vi "AD（V3.2）150M.vi"(2 "量程选择":u32, 8 "N-length":dbl, 9 "M-length":dbl, 10 "hDevice":i32, 11 "待读取数据长度":u32) -> (0 "幅频谱":dbl[](graph), 1 "时域谱":dbl[](graph), 3 "hDevice out":i32)   [LabVIEW 2016]
uses:
  <vilib>/Analysis/2dsp.llb/Real FFT.vi
  <vilib>/Analysis/NI_AALPro.lvlib
  E:/PCI8552B/Driver/INF/Win32&Win64/amd64/PCI8552B_32.dll
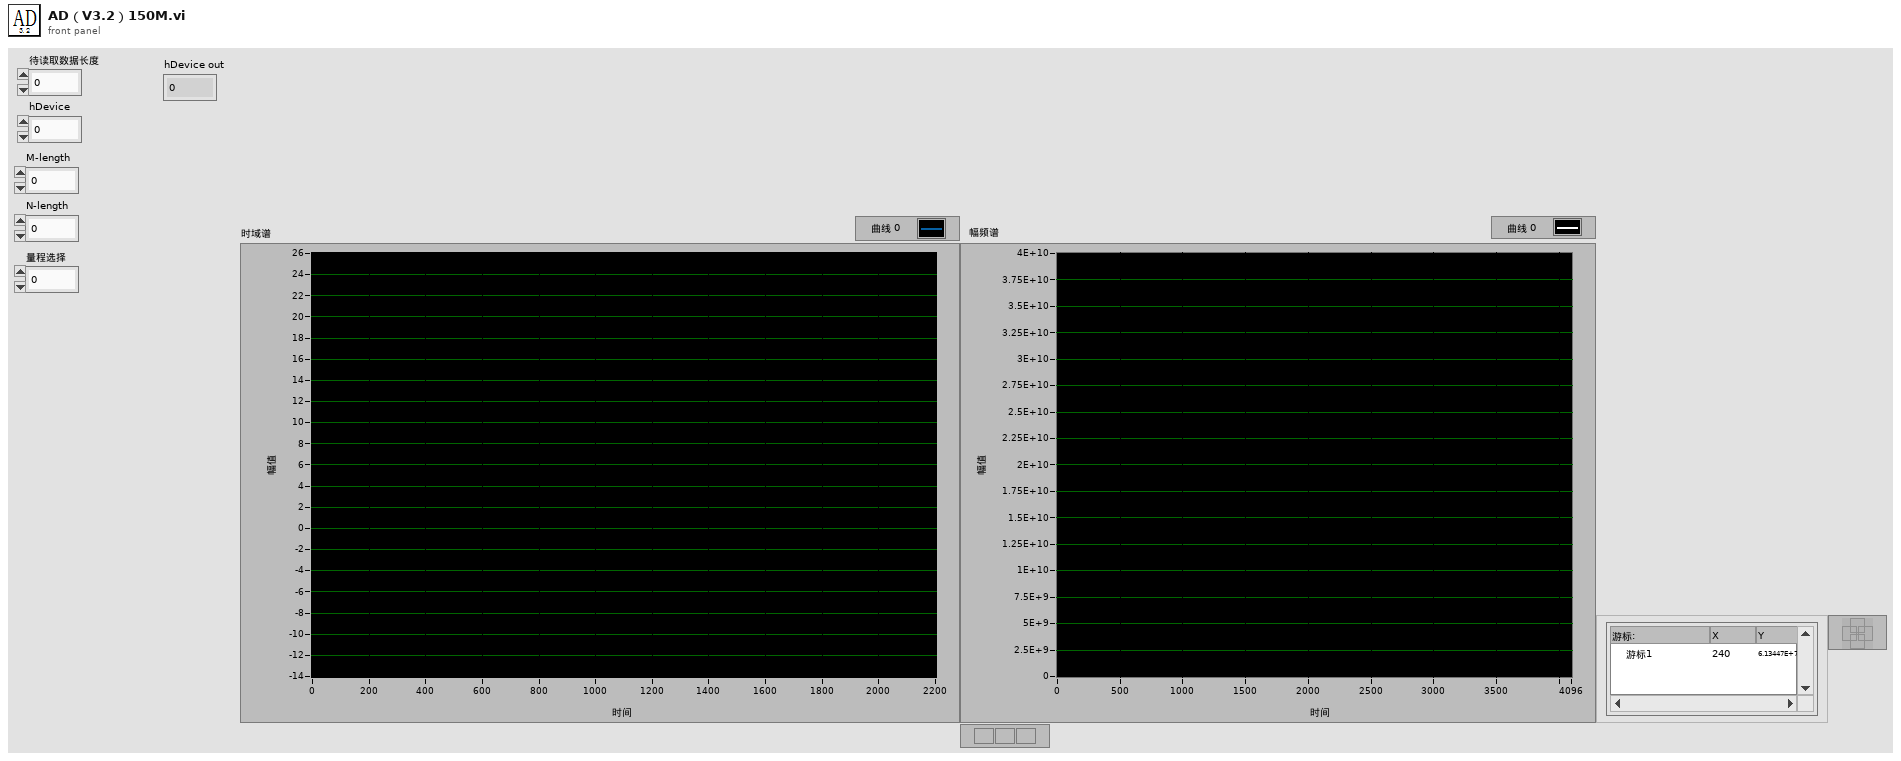
[diagram p1: front panel]
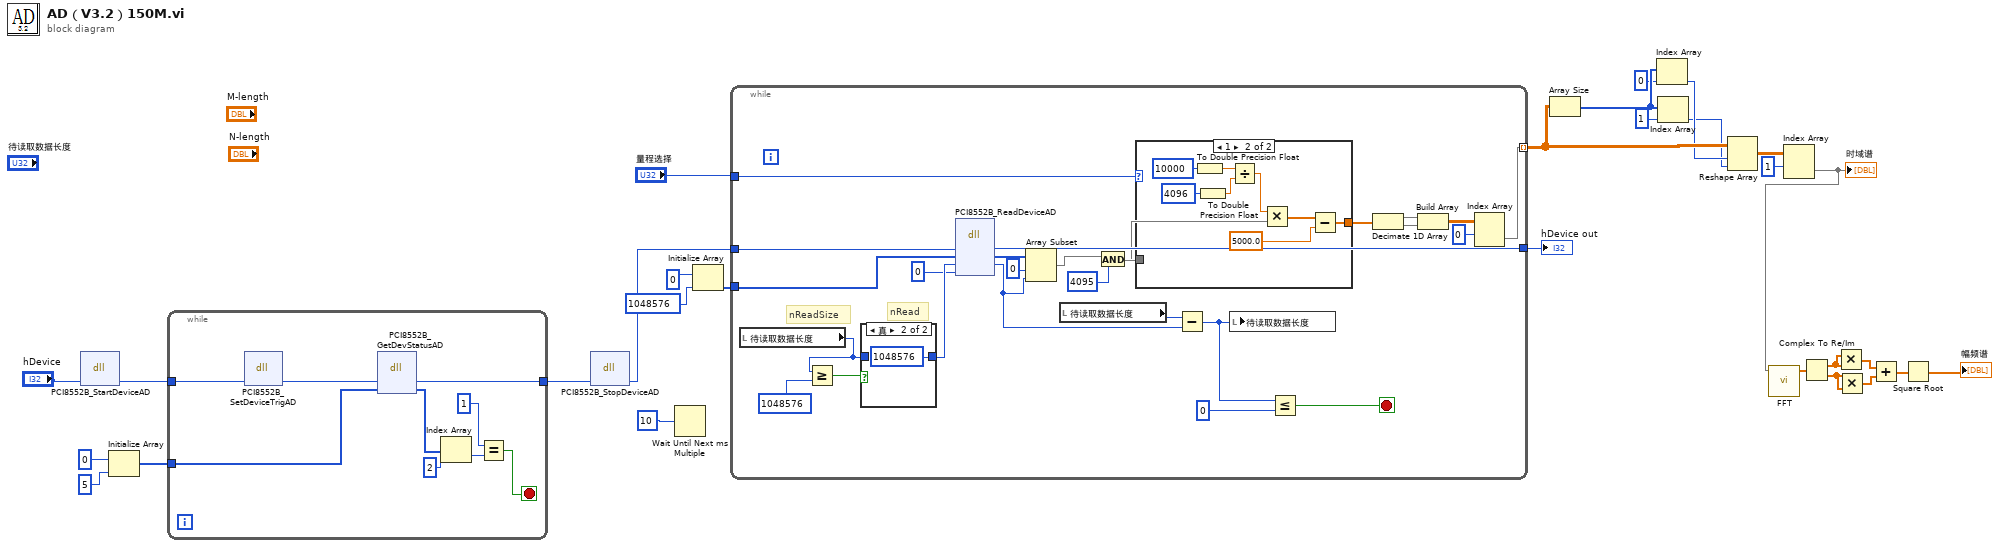
[diagram p0: block diagram]
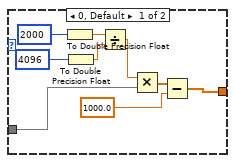
[diagram p2: hidden frame]
diagram:
  n1 = dll-call lib="E:/PCI8552B/Driver/INF/Win32&Win64/amd64/PCI8552B_32.dll" fn="PCI8552B_StartDeviceAD" label="StartDeviceAD"("hDevice"="hDevice") -> ("hDevice"=w24:i32)  [unwired: 4 in, 2 out]
  n2 = Initialize Array(0, 5) -> (w28:i32[])
  n3 = while {
    tunnel: w24 -> [w34]
    tunnel: w28 -> [w38]
    tunnel: [w32] -> w25
    stop <- w31 stop-if-true
    n4 = dll-call lib="E:/PCI8552B/Driver/INF/Win32&Win64/amd64/PCI8552B_32.dll" fn="PCI8552B_SetDeviceTrigAD" label="SetDeviceTrigAD"("hDevice"=w34) -> ("hDevice"=w33:i32)  [unwired: 4 in, 2 out]
    n5 = dll-call lib="E:/PCI8552B/Driver/INF/Win32&Win64/amd64/PCI8552B_32.dll" fn="PCI8552B_GetDevStatusAD" label="GetDevStatusAD"("hDevice"=w33, "ADStatus"=w38) -> ("hDevice"=w32:i32, "ADStatus"=w35:i32[])  [unwired: 4 in, 2 out]
    n6 = Index Array(array=w35, index=2) -> (element=w30:i32)
    n7 = Equal?(x=1, y=w30) -> (x = y?=w31:bool)
  }
  n8 = dll-call lib="E:/PCI8552B/Driver/INF/Win32&Win64/amd64/PCI8552B_32.dll" fn="PCI8552B_StopDeviceAD" label="StopDeviceAD"("hDevice"=w25) -> ("hDevice"=w20:i32)  [unwired: 4 in, 2 out]
  n9 = Wait Until Next ms Multiple(millisecond multiple=u32 10) -> ()  [unwired: 1 out]
  n10 = Initialize Array(u16 0 ("y"), 1048576 ("y")) -> (w21:u16[])
  n11 = while {
    tunnel: w20 -> [w63]
    tunnel: [w62] -> w10
    tunnel: w21 -> [w61]
    tunnel: "量程选择" -> [w51]
    tunnel: [w39] -> w9 mode=indexing
    stop <- w42 stop-if-true
    # "nReadSize"
    # "nRead"
    n12 = local read "待读取数据长度"() -> (w57:u32)
    n13 = Greater Or Equal?(x=w57, y=1048576 ("millisecond multiple")) -> (x >= y?=w59:bool)
    n14 = case shown="真" w59 {
      tunnel: [w82 1048576 ("millisecond multiple")] -> w54
      tunnel: w57 -> [w82 _]
      frame False {
      }
      frame True {
      }
    }
    n15 = dll-call lib="E:/PCI8552B/Driver/INF/Win32&Win64/amd64/PCI8552B_32.dll" fn="PCI8552B_ReadDeviceAD" label="ReadDeviceAD"("hDevice"=w63, "pADBuffer"=w61, "nReadSizeWords"=w54, "nRetSizeWords"=0) -> ("hDevice"=w62:i32, "pADBuffer"=w48:u16[], "nReadSizeWords"=w45:u32)  [unwired: 5 in, 2 out]
    n16 = Array Subset(array=w48, index=0 ("索引"), length=w45) -> (w47:u16[])
    n17 = local read "待读取数据长度"() -> (w56:u32)
    n18 = And(x=w47, y=u16 4095) -> (x .and. y?=w52:u16[])
    n19 = case shown="1" w51 {
      tunnel: w52 -> [w71 w76]
      tunnel: [w64 w75] -> w50
      frame 0, Default {
        n20 = To Double Precision Float(number=2000 ("x")) -> (double precision float=w67:dbl)
        n21 = To Double Precision Float(number=4096) -> (double precision float=w66:dbl)
        n22 = Divide(x=w67, y=w66) -> (x/y=w72:dbl)
        n23 = Multiply(x=w72, y=w71) -> (x*y=w70:dbl[])
        n24 = Subtract(x=w70, y=1000.0) -> (x-y=w64:dbl[])
      }
      frame 1 {
        n25 = To Double Precision Float(number=10000 ("x")) -> (double precision float=w74:dbl)
        n26 = To Double Precision Float(number=4096) -> (double precision float=w78:dbl)
        n27 = Divide(x=w74, y=w78) -> (x/y=w81:dbl)
        n28 = Multiply(x=w81, y=w76) -> (x*y=w80:dbl[])
        n29 = Subtract(x=w80, y=5000.0) -> (x-y=w75:dbl[])
      }
    }
    n30 = Subtract(x=w56, y=w45) -> (x-y=w55:u32)
    n31 = local write "待读取数据长度"(w55) -> ()
    n32 = Less Or Equal?(x=w55, y=0) -> (x <= y?=w42:bool)
    n33 = Decimate 1D Array(w50) -> (w44:dbl[], w43:dbl[])
    n34 = Build Array(w44, w43) -> (w40:dbl[][])
    n35 = Index Array(array=w40, index (row)=0 ("索引")) -> (element=w39:dbl[])  [unwired: 1 in]
  }
  "hDevice out" <- w10
  n36 = Array Size(array=w9) -> (size(s)=w8:i32[])
  n37 = Index Array(array=w8, index=0 ("索引")) -> (element=w5:i32)
  n38 = Index Array(array=w8, index=1 ("索引")) -> (element=w4:i32)
  n39 = Reshape Array(w9, w5, w4) -> (w3:dbl[][])
  n40 = Index Array(array=w3, index (row)=1 ("索引 (行)")) -> (element=w1:dbl[])  [unwired: 1 in]
  "时域谱" <- w1
  n41 = call-poly <vilib>:"FFT.vi"("X"=w1) -> ("FFT {X}"=w13:cdb[])  [unwired: 9 in, 1 out]
  n42 = Complex To Re/Im(x + iy=w13) -> (x=w14:dbl[], y=w15:dbl[])
  n43 = Multiply(x=w14, y=w14) -> (x*y=w16:dbl[])
  n44 = Multiply(x=w15, y=w15) -> (x*y=w17:dbl[])
  n45 = Add(x=w16, y=w17) -> (x+y=w18:dbl[])
  n46 = Square Root(x=w18) -> (sqrt(x)=→"幅频谱":dbl[])
